vi "testGetShot.vi"() -> ()   [LabVIEW 2011]
panel:
  out "Shot":i32
  out "Array":dbl[](array[numeric])
  in  "Start Event":string="Shot_Init"
  out "Connect status":i32
  in  "Host":string="shanghai.ph.utexas.edu"
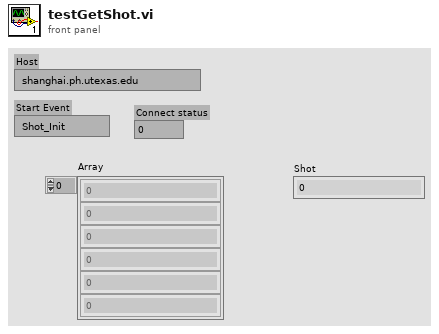
[diagram p1: front panel]
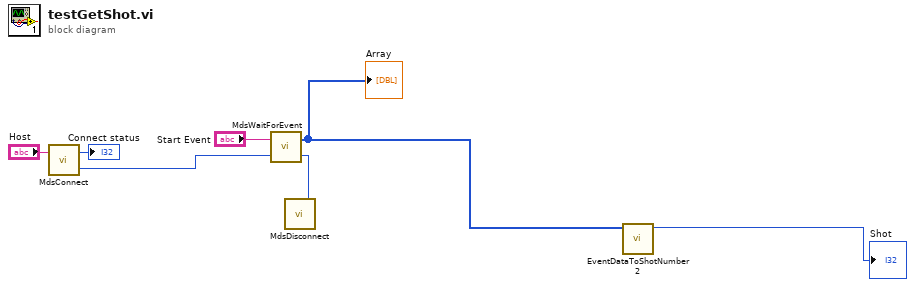
[diagram p0: block diagram]
diagram:
  n1 = call "MdsConnect.vi"("Host"="Host") -> ("FlowControlOut"=w4:i32, "Status"=→"Connect status":i32)  [unwired: 1 in]
  n2 = call "MdsWaitForEvent.vi"("FlowControlIn"=w4, "Event"="Start Event") -> ("FlowControlOut"=w3:i32, "EventData"=w2:u8[])
  "Array" <- w2
  n3 = call "MdsDisconnect.vi"("FlowControlIn"=w3) -> ()  [unwired: 1 out]
  n4 = call "EventDataToShotNumber2.vi"("EventDataIn"=w2) -> ("ShotNumberOut"=→"Shot":i32)  [unwired: 10 in]
